vi "Aggregate Assertion Results.vi"(10 "Assertion Result":refnum<class "Assertion Result.lvclass">, 11 "Method Result In":refnum<class "Method Result.lvclass">) -> (3 "Method Result Out":refnum<class "Method Result.lvclass">)   [LabVIEW 2020, in "Method Result.lvclass"]
uses:
  Method Result.lvclass
  Assertion Result/Assertion Result.lvclass
  Assertion Result/Assertion Result.lvclass/Assertion Result.ctl
  Method Result.lvclass/Method Result.ctl
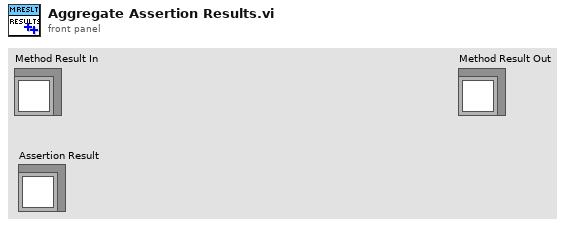
[diagram p1: front panel]
types:
  T1 = typedef "Assertion Result.lvclass/Status.ctl" = enum16{"Pass", "Fail", "Error", "Skipped", "Setup Error", "Broken", "Teardown Error"}
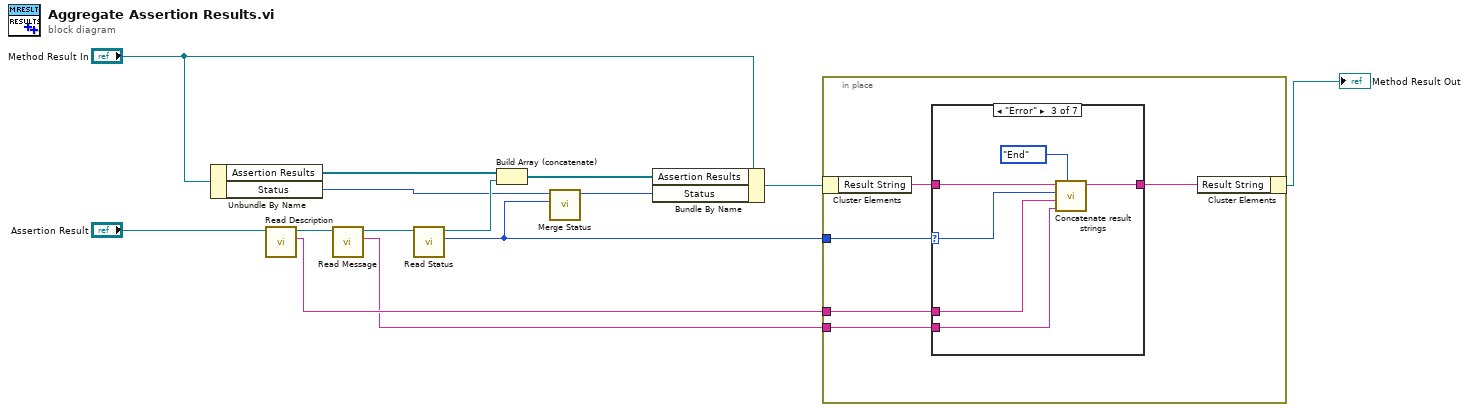
[diagram p0: block diagram]
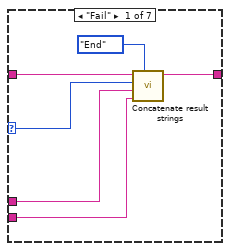
[diagram p2: hidden frame]
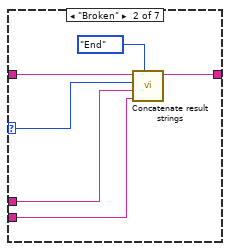
[diagram p3: hidden frame]
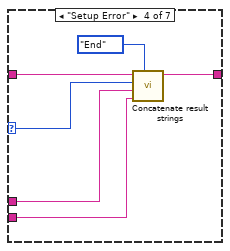
[diagram p4: hidden frame]
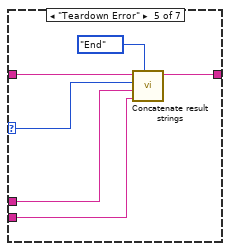
[diagram p5: hidden frame]
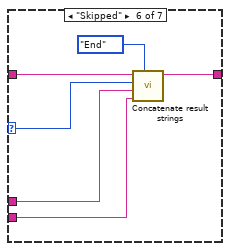
[diagram p6: hidden frame]
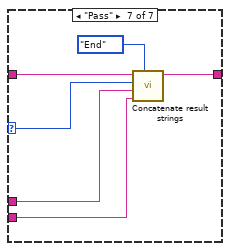
[diagram p7: hidden frame]
diagram:
  n1 = Unbundle By Name("Method Result In") -> ("Assertion Results"=w13:refnum<class "Assertion Result.lvclass">[], "Status"=w5:T1)
  n2 = call "Read Description.vi"("Assertion Result In"="Assertion Result") -> ("Description"=w10:string, "Assertion Result Out"=w8:refnum<class "Assertion Result.lvclass">)  [unwired: 9 in]
  n3 = call "Read Message.vi"("Assertion Result In"=w8) -> ("Message"=w6:string, "Assertion Result Out"=w1:refnum<class "Assertion Result.lvclass">)  [unwired: 9 in]
  n4 = call "Read Status.vi"("Assertion Result In"=w1) -> ("Status"=w3:T1, "Assertion Result Out"=w11:refnum<class "Assertion Result.lvclass">)  [unwired: 9 in]
  n5 = Build Array (concatenate)(w13, w11) -> (w12:refnum<class "Assertion Result.lvclass">[])
  n6 = call "Merge Status.vi"("New"=w3, "Current"=w5) -> ("Merged"=w4:T1)  [unwired: 8 in, 1 out]
  n7 = Bundle By Name(cluster="Method Result In", "Assertion Results"=w12, "Status"=w4) -> (w7:refnum<class "Method Result.lvclass">)
  n8 = in-place {
    in-place-border: w10 -> [w19]
    in-place-border: w3 -> [w16]
    in-place-border: w6 -> [w15]
    n9 = in-place-cluster #1(w7) -> ("Result String"=w18:string)
    n10 = case shown="\"Error\"" w16 {
      selector: w16 -> [w22 w28 w34 w40 w46 w52 w58]
      tunnel: w19 -> [w25 w31 w37 w43 w49 w55 w61]
      tunnel: w18 -> [w24 w30 w36 w42 w48 w54 w60]
      tunnel: [w23 w29 w35 w41 w47 w53 w59] -> w17
      tunnel: w15 -> [w21 w27 w33 w39 w45 w51 w57]
      frame "Fail" {
        n11 = call "Concatenate result strings.vi"("Location"=enum16{"Start", "End"}."End", "Message"=w21, "Description"=w25, "Status"=w22, "Input String"=w24) -> ("Output String"=w23:string)  [unwired: 6 in]
      }
      frame "Broken" {
        n12 = call "Concatenate result strings.vi"("Location"=enum16{"Start", "End"}."End", "Message"=w27, "Description"=w31, "Status"=w28, "Input String"=w30) -> ("Output String"=w29:string)  [unwired: 6 in]
      }
      frame "Error" {
        n13 = call "Concatenate result strings.vi"("Location"=enum16{"Start", "End"}."End", "Message"=w33, "Description"=w37, "Status"=w34, "Input String"=w36) -> ("Output String"=w35:string)  [unwired: 6 in]
      }
      frame "Setup Error" {
        n14 = call "Concatenate result strings.vi"("Location"=enum16{"Start", "End"}."End", "Message"=w39, "Description"=w43, "Status"=w40, "Input String"=w42) -> ("Output String"=w41:string)  [unwired: 6 in]
      }
      frame "Teardown Error" {
        n15 = call "Concatenate result strings.vi"("Location"=enum16{"Start", "End"}."End", "Message"=w45, "Description"=w49, "Status"=w46, "Input String"=w48) -> ("Output String"=w47:string)  [unwired: 6 in]
      }
      frame "Skipped" {
        n16 = call "Concatenate result strings.vi"("Location"=enum16{"Start", "End"}."End", "Message"=w51, "Description"=w55, "Status"=w52, "Input String"=w54) -> ("Output String"=w53:string)  [unwired: 6 in]
      }
      frame "Pass" {
        n17 = call "Concatenate result strings.vi"("Location"=enum16{"Start", "End"}."End", "Message"=w57, "Description"=w61, "Status"=w58, "Input String"=w60) -> ("Output String"=w59:string)  [unwired: 6 in]
      }
    }
    n18 = in-place-cluster #1("Result String"=w17) -> (→"Method Result Out":refnum<class "Method Result.lvclass">)
  }
